vi "LoggerDaemon.vi"(6 "Write delay (ms)":u32=1000, 8 "error in (no error)":errorcluster, 9 "Stop Cmd Reference":refnum<data-value>, 10 "Log Message Queue":refnum<queue>, 11 "File path":path) -> (0 "error out":errorcluster)   [LabVIEW 2011, in "Logger.lvclass"]
doc: "Daemon (running in the background) which consistently checks the internal queue for new data to log. When there is some, it writes to the text file.\n\nJared Kirschner, 2012."
uses:
  Logger.lvclass
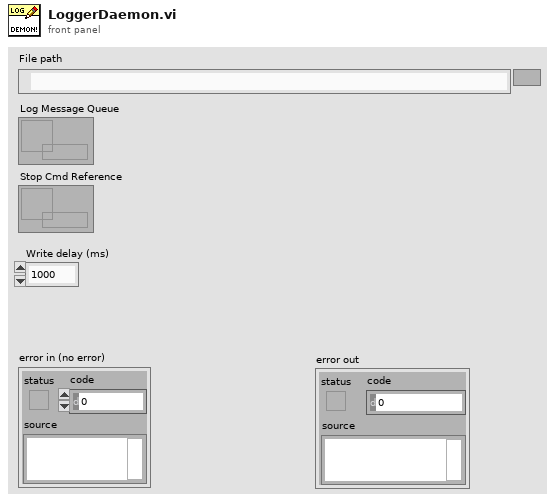
[diagram p1: front panel]
types:
  T1 = enum16{"open", "replace", "create", "open or create", "replace or create", "replace or create with confirmation"}
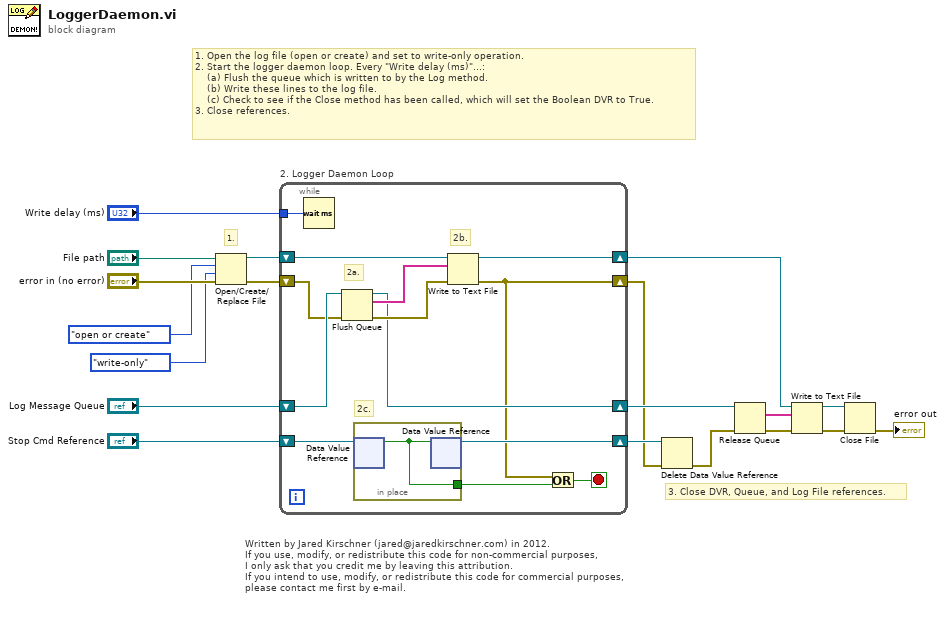
[diagram p0: block diagram]
diagram:
  # "Written by Jared Kirschner (jared@jaredkirschner.com) in 2012.\nIf you use, modify, or redistribute this code for non-commercial purposes,\nI only ask that you credit me by leaving this attribution.\nIf you intend to use, modify, or redistribute this code for commercial purposes,\nplease contact me first by e-mail."
  # "3. Close DVR, Queue, and Log File references."
  # "1."
  # "1. Open the log file (open or create) and set to write-only operation.\n2. Start the logger daemon loop. Every \"Write delay (ms)\"...:\n    (a) Flush the queue which is written to by the Log method.\n    (b) Write these lines to the log file.\n    (c) Check to see if the Close method has been called, which will set the Boolean DVR to True.\n3. Close references."
  n1 = Open/Create/Replace File(file path (use dialog)="File path", error in="error in (no error)", operation (0:open)=T1."open or create", access (0:read/write)=enum16{"read/write", "read-only", "write-only"}."write-only") -> (refnum out=w10:refnum<file>, error out=w9:errorcluster)  [unwired: 2 in, 1 out]
  n2 = while "2. Logger Daemon Loop" {
    shift-right: [w31] -> w18
    shift-left: "Stop Cmd Reference" -> [w32]
    tunnel: "Write delay (ms)" -> [w30]
    shift-right: [w23] -> w15
    shift-left: "Log Message Queue" -> [w29]
    shift-right: [w24] -> w6
    shift-left: w10 -> [w27]
    shift-right: [w20] -> w2
    shift-left: w9 -> [w28]
    stop <- w21 stop-if-true
    # "2c."
    # "2b."
    # "2a."
    n3 = Wait (ms)(milliseconds to wait=w30) -> ()  [unwired: 1 out]
    n4 = Flush Queue(queue=w29, error in (no error)=w28) -> (queue out=w23:refnum<queue>, remaining elements=w26:string[], error out=w25:errorcluster)
    n5 = in-place {
      in-place-border: [w33] -> w22
      n6 = in-place-dvr #1(w32) -> (w33:bool)  [unwired: 1 out]
      n7 = in-place-dvr #1(w33) -> (w31:refnum<data-value>)  [unwired: 1 out]
    }
    n8 = Write to Text File(file (use dialog)=w27, text=w26, error in=w25) -> (refnum out=w24:refnum<file>, error out=w20:errorcluster)  [unwired: 1 in, 1 out]
    n9 = Or(x=w20, y=w22) -> (x .or. y?=w21:bool)
  }
  n10 = Delete Data Value Reference(data value reference=w18, error in=w2) -> (error out=w1:errorcluster)  [unwired: 1 out]
  n11 = Release Queue(queue=w15, error in (no error)=w1) -> (remaining elements=w7:string[], error out=w8:errorcluster)  [unwired: 1 in, 1 out]
  n12 = Write to Text File(file (use dialog)=w6, text=w7, error in=w8) -> (refnum out=w5:refnum<file>, error out=w4:errorcluster)  [unwired: 1 in, 1 out]
  n13 = Close File(refnum=w5, error in=w4) -> (error out=→"error out":errorcluster)  [unwired: 1 out]
